vi "Count Digital Pulses 1000ms.vi"() -> ()   [LabVIEW 2020]
uses:
  <vilib>/DAQmx/read.llb/DAQmx Read (Counter U32 1Chan 1Samp).vi
  <vilib>/DAQmx/create/channels.llb/DAQmx Create Channel (CI-Count Edges).vi
  <vilib>/DAQmx/miscellaneous.llb/DAQmx Fill In Error Info.vi
panel:
  out "Numeric":dbl
  in  "stop":bool
  out "Counts":dbl
  in  "edge":i32(ring)=10280 items=["Rising"=10280, "Falling"=10171]
  in  "count direction":i32(ring)=10128 items=["Count Up"=10128, "Count Down"=10124, "Externally Controlled"=10326]
  in  "initial count":u32
  in  "DAQmx Physical Channel":tag
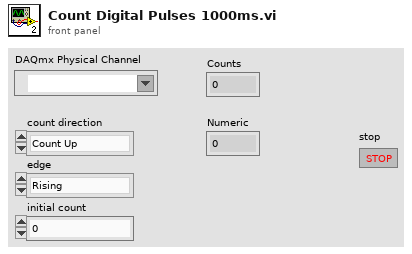
[diagram p1: front panel]
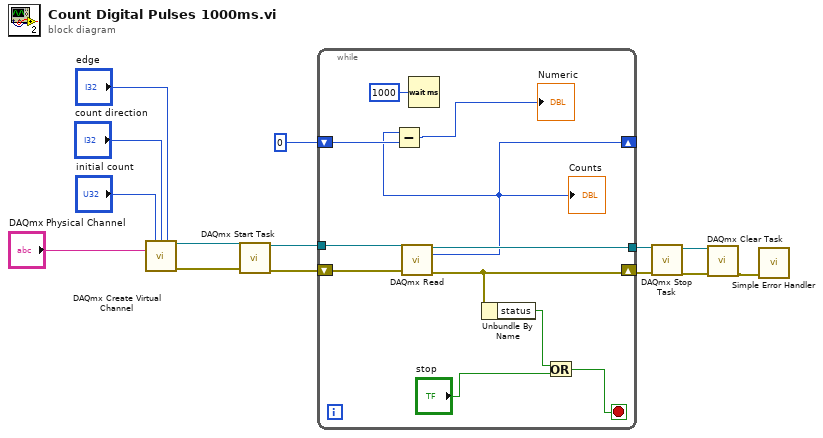
[diagram p0: block diagram]
diagram:
  n1 = call-poly <vilib>:"DAQmx Create Virtual Channel.vi"("initial count"="initial count", "count direction"="count direction", "edge"="edge", "counter"="DAQmx Physical Channel") -> ("task out"=w11:refnum<k21>, "error out"=w10:errorcluster)  [unwired: 10 in]
  n2 = call <vilib>:"DAQmx Start Task.vi"("task/channels in"=w11, "error in"=w10) -> ("task out"=w9:refnum<k21>, "error out"=w8:errorcluster)  [unwired: 12 in]
  n3 = while {
    tunnel: w9 -> [w25]
    tunnel: [w22] -> w7
    shift-right: [w21] -> w6
    shift-left: w8 -> [w24]
    shift-right: [w16] -> _
    shift-left: 0 -> [w17]
    stop <- w18 stop-if-true
    n4 = call-poly <vilib>:"DAQmx Read.vi"("task/channels in"=w25, "error in"=w24) -> ("task out"=w22:refnum<k21>, "data"=w16:u32, "error out"=w21:errorcluster)  [unwired: 11 in]
    "Counts" <- w16
    n5 = Subtract(x=w16, y=w17) -> (x-y=→"Numeric":u32)
    n6 = Wait (ms)(milliseconds to wait=u32 1000) -> ()  [unwired: 1 out]
    n7 = Unbundle By Name(w21) -> ("status"=w19:bool)
    n8 = Or(x=w19, y="stop") -> (x .or. y?=w18:bool)
  }
  n9 = call <vilib>:"DAQmx Stop Task.vi"("task/channels in"=w7, "error in"=w6) -> ("task out"=w5:refnum<k21>, "error out"=w4:errorcluster)  [unwired: 12 in]
  n10 = call <vilib>:"DAQmx Clear Task.vi"("task in"=w5, "error in"=w4) -> ("error out"=w3:errorcluster)  [unwired: 13 in]
  n11 = call <vilib>:"Simple Error Handler.vi"("error in (no error)"=w3) -> ()  [unwired: 4 in, 5 out]
